vi "DISP_WIND_TITL_DATA.vi"(0 "VISA IN":refnum<visa-resource-name>, 1 "Title":string, 5 "error in":errorcluster, 7 "Window":i32=1) -> (14 "VISA Out":refnum<visa-resource-name>, 19 "error out":errorcluster)   [LabVIEW 2018, in "PNA-X.lvlib"]
doc: "DISPlay:WINDow<wnum>:TITLe:DATA <string> \n(Read-Write) Sets data in the window title area. The title is turned ON and OFF with \nDISP:WIND:TITL:STAT OFF. \nParameters \n<wnum> Any existing window number. If unspecified, value is set to 1. \n<string> Title to be displayed. Any characters, enclosed with quotes. If the title string \nexceeds 50 characters, an error will be generated and the title not accepted. \nNewer entries replace (not append) older entries. \nExamples DISP:WIND:TITL:DATA 'hello' \ndisplay:window2:title:data 'hello' \nQuery Syntax DISPlay:WINDow<wnum>:TITLe:DATA? \nReturn Type String \nDefault NA"
uses:
  PNA-X.lvlib
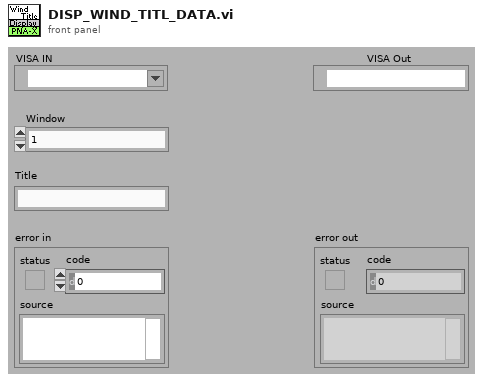
[diagram p1: front panel]
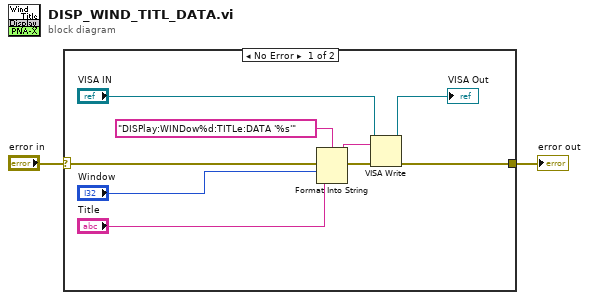
[diagram p0: block diagram]
diagram:
  n1 = case shown="No Error" "error in" {
    selector: "error in" -> [w11 w12]
    tunnel: [w6 w12] -> w1
    frame No Error {
      n2 = Format Into String(format string="DISPlay:WINDow%d:TITLe:DATA '%s'" ("Cmdline"), error in=w11, "Window", "Title") -> (resulting string=w9:string, error out=w10:errorcluster)  [unwired: 1 in]
      n3 = VISA Write(VISA resource name="VISA IN", write buffer=w9, error in (no error)=w10) -> (VISA resource name out=→"VISA Out":refnum<visa-resource-name>, error out=w6:errorcluster)  [unwired: 1 out]
    }
    frame Error {
    }
  }
  "error out" <- w1
